vi "NewNYStyleClamPizza.vi"(8 "error in (no error)":errorcluster) -> (0 "error out":errorcluster, 3 "NYStyleClamPizza":refnum<class "NYStyleClamPizza.lvclass">)   [LabVIEW 2020, in "FactoryMethod.lvlib" / "PizzaFactoryMethod.lvlib" / "NYStyleClamPizza.lvclass"]
uses:
  NYStyleClamPizza.lvclass
  NYStyleClamPizza.lvclass/NYStyleClamPizza.ctl
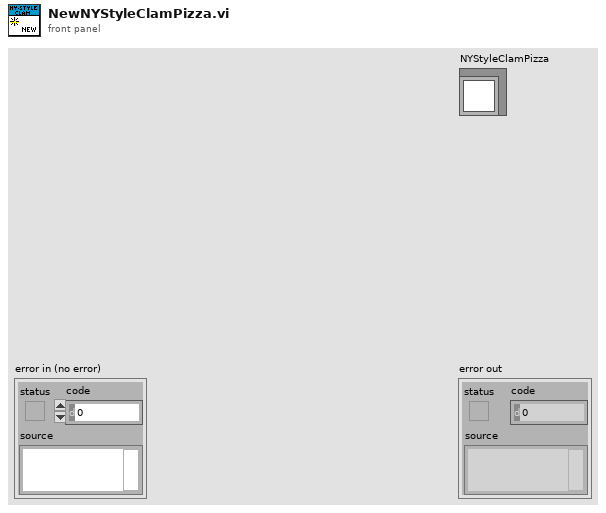
[diagram p1: front panel]
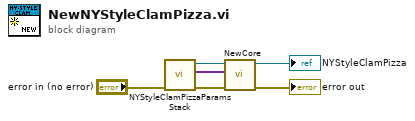
[diagram p0: block diagram]
diagram:
  n1 = call "NYStyleClamPizzaParamsStack.vi"("error iN"="error in (no error)") -> ("error out"=w6:errorcluster, "HierarchyParams"=w5:variant[], "NYStyleClamPizza"=w1:refnum<class "NYStyleClamPizza.lvclass">)  [unwired: 8 in]
  n2 = call-dynamic "NewCore.vi"("error in (no error)"=w6, "ParamsArray"=w5, "NYStyleClamPizza"=w1) -> ("error out"=→"error out":errorcluster, "NYStyleClamPizza"=→"NYStyleClamPizza":refnum<class "NYStyleClamPizza.lvclass">)  [unwired: 7 in]
